vi "fpga_DAC_sine_and_ADC.vi"() -> ()   [LabVIEW 2018]
uses:
  <vilib>/rvi/FXPMathLib/FxpSinAndCos/subVIs/nifxpmath_SinAndCos_SimConfig.ctl
  <vilib>/rvi/Emulation/niFpgaGetClockAttributes.vi
  <vilib>/rvi/Emulation/niFpgaSctlEmulationGetInTimedLoop.vi
  <vilib>/rvi/Emulation/niFpgaEmulationReportErrorSimple.vi
  <vilib>/rvi/eio/common/nirviEmuTemplateMethod_errors.vi
  <vilib>/rvi/FXPMathLib/FxpSinAndCos/simVIs/DllFxpSinAndCosTemp_sub.vi
  <vilib>/rvi/Emulation/niFpgaCriticalErrorInLSC.vi
  <vilib>/eio/EIONode/EIONode.xnode
  <vilib>/rvi/FXPMathLib/FxpSinAndCos/XNode/nifxpmath_SinAndCos.xnode
panel:
  in  "Stop":bool
  in  "delay (us)":u32=40000
  out "ADC CH1 read":bool[](array[boolean])
  in  "ADC CH1 write":bool[](array[boolean])=[FALSE, FALSE, FALSE, FALSE, FALSE, TRUE, FALSE, FALSE, FALSE, FALSE, FALSE, FALSE, FALSE, FALSE, FALSE, FALSE]
  in  "offset (V)":fxp<+/-,9,5>
  in  "amplitude (V)":fxp<+/-,9,5>=2.5
  in  "datapoints/cycle":u16=100
  out "DAC 1 write":bool[](array[boolean])=[FALSE, TRUE, TRUE, TRUE, FALSE, FALSE, TRUE, TRUE, TRUE, TRUE, FALSE, TRUE, FALSE, FALSE, TRUE, TRUE]
  # "+/-10 V range"
  # "for 100 datapoints per sine cycle,"
  # "at 40000 us delay, sine frequency will be 10 Hz\nand ADC will be sampled at 1 kHz. This also will be loop rate of the program"
  # "at 320 us delay, the program runs at its max loop rate of 125 kHz. \nbut the gain at this frequency is very low for the system, it hardly moves"
  # "at 16000 us delay, sine frequency will be 25 Hz, (resonant frequency of the system)\nwith an amplitude of 1, cap probe's full range of +/- 10 V could be reached, since Q factor\nis high at resonance\nADC will be sampled at 2.5 kHz. This also will be loop rate of the program"
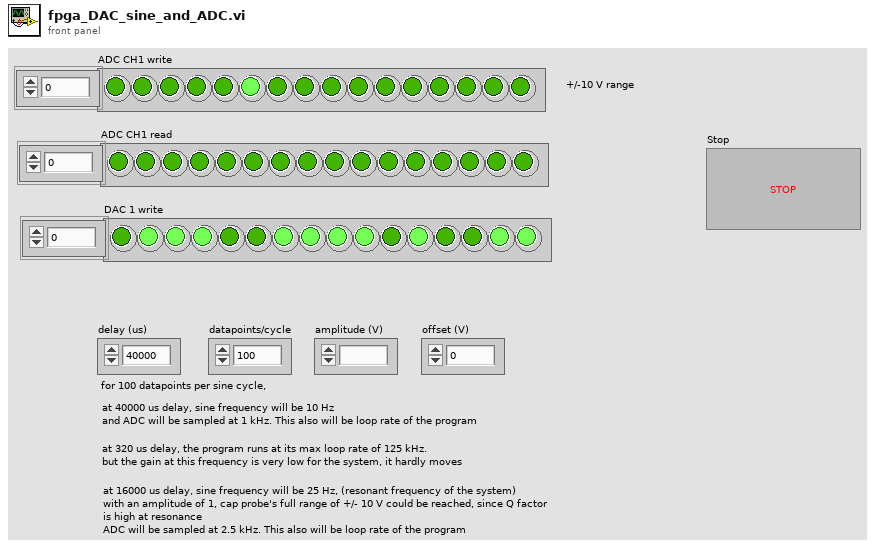
[diagram p1: front panel]
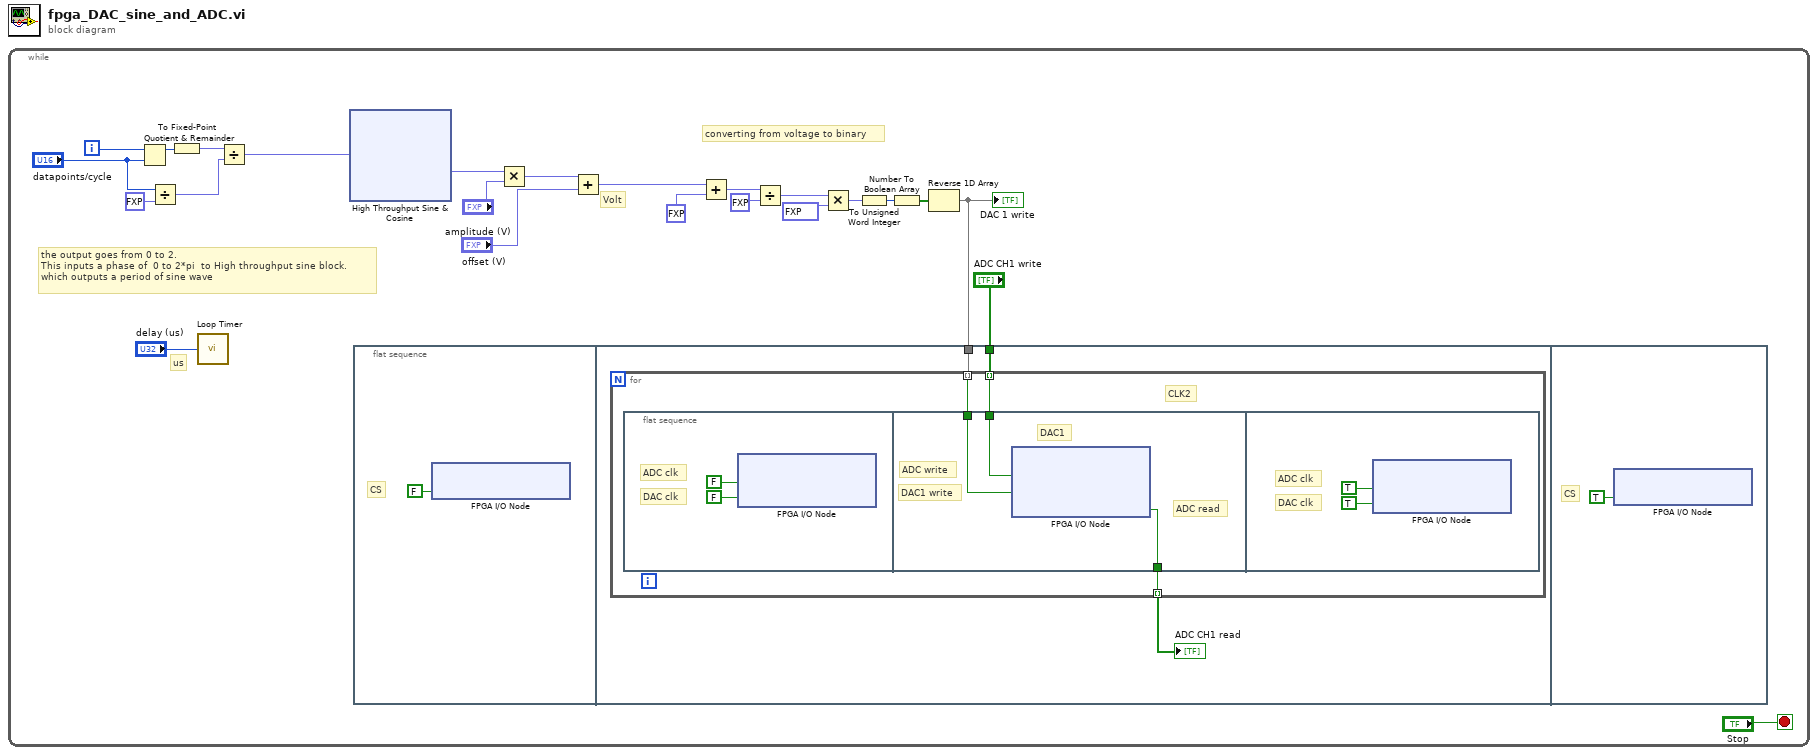
[diagram p0: block diagram]
diagram:
  n1 = while {
    i -> [w13]
    stop <- "Stop" stop-if-true
    # "converting from voltage to binary"
    # "us"
    # "Volt"
    # "the output goes from 0 to 2.\nThis inputs a phase of  0 to 2*pi  to High throughput sine block.\nwhich outputs a period of sine wave"
    n2 = Quotient & Remainder(x=w13, y="datapoints/cycle") -> (x-y*floor(x/y)=w12:i32)  [unwired: 1 out]
    n3 = Divide(x="datapoints/cycle", y=fxp<+,1,2> 2.0) -> (x/y=w4:fxp<+,17,15>)
    n4 = To Fixed-Point(number=w12) -> (fixed-point=w6:fxp<+/-,16,12>)  [unwired: 1 in]
    n5 = call "Loop Timer"("Count(Ticks)"="delay (us)") -> ()  [unwired: 1 out]
    n6 = Divide(x=w6, y=w4) -> (x/y=w11:fxp<+/-,33,14>)
    n7 = xnode "High Throughput Sine & Cosine"("x (pi)"=w11) -> ("sin(x)"=w10:fxp<+/-,16,2>)  [unwired: 1 out]
    n8 = flat-sequence {
      tunnel: w17 -> [w58]
      tunnel: "ADC CH1 write" -> [w57]
      frame #0 {
        # "CS"
        n9 = xnode "FPGA I/O Node"("ConnectorA/DIO4"=FALSE) -> ()  [unwired: 1 in, 1 out]
      }
      frame #1 {
        n10 = for {
          tunnel: w58 -> [w61] mode=indexing
          tunnel: w57 -> [w60] mode=indexing
          tunnel: [w59] -> w56 mode=indexing
          # "CLK2"
          n11 = flat-sequence {
            tunnel: w61 -> [w66]
            tunnel: w60 -> [w65]
            tunnel: [w64] -> w59
            frame #0 {
              # "DAC clk"
              # "ADC clk"
              n12 = xnode "FPGA I/O Node"("ConnectorA/DIO3"=FALSE, "ConnectorA/DIO5"=FALSE) -> ()  [unwired: 2 in, 2 out]
            }
            frame #1 {
              # "ADC read"
              # "DAC1 write"
              # "ADC write"
              # "DAC1"
              n13 = xnode "FPGA I/O Node"("ConnectorA/DIO2"=w65, "ConnectorA/DIO6"=w66) -> ("ConnectorA/DIO1"=w64:bool)  [unwired: 3 in, 3 out]
            }
            frame #2 {
              # "DAC clk"
              # "ADC clk"
              n14 = xnode "FPGA I/O Node"("ConnectorA/DIO3"=TRUE, "ConnectorA/DIO5"=TRUE) -> ()  [unwired: 2 in, 2 out]
            }
          }
        }
        "ADC CH1 read" <- w56
      }
      frame #2 {
        # "CS"
        n15 = xnode "FPGA I/O Node"("ConnectorA/DIO4"=TRUE) -> ()  [unwired: 1 in, 1 out]
      }
    }
    n16 = Multiply(x=w10, y="amplitude (V)") -> (x*y=w15:fxp<+/-,25,7>)
    n17 = Add(x=w15, y="offset (V)") -> (x+y=w9:fxp<+/-,25,7>)
    n18 = Add(x=w9, y=fxp<+,3,4> 10.0) -> (x+y=w22:fxp<+/-,25,7>)
    n19 = Divide(x=w22, y=fxp<+,3,5> 20.0) -> (x/y=w8:fxp<+/-,26,3>)
    n20 = Multiply(x=w8, y=fxp<+,16,16> 65535.0) -> (x*y=w7:fxp<+/-,42,19>)
    n21 = To Unsigned Word Integer(number=w7) -> (unsigned 16bit integer=w20:u16)
    n22 = Number To Boolean Array(number=w20) -> (Boolean array=w19:bool[])
    n23 = Reverse 1D Array(array=w19) -> (reversed array=w17:bool[])
    "DAC 1 write" <- w17
  }
